vi "String.vi"() -> (0 "error out":errorcluster, 3 "Passed?":bool)   [LabVIEW 2009]
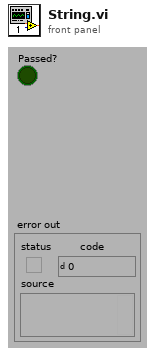
[diagram p1: front panel]
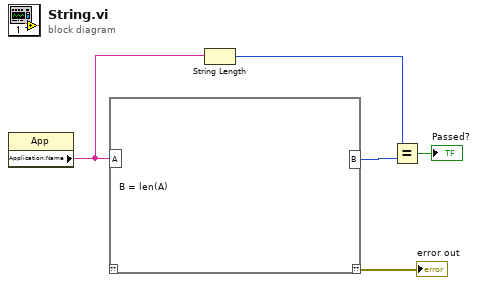
[diagram p0: block diagram]
diagram:
  n1 = property class="App"() -> ("Application:Name"=w3:string)  [unwired: 2 in, 2 out]
  n2 = script code="B = len(A)"("A"=w3) -> ("??"=→"error out":errorcluster, "B"=w1:i32)  [unwired: 1 in]
  n3 = String Length(string=w3) -> (length=w2:i32)
  n4 = Equal?(x=w2, y=w1) -> (x = y?=→"Passed?":bool)
